vi "parse_binaries.vi"(4 "error in":errorcluster) -> (0 "error out":errorcluster)   [LabVIEW 2019]
doc: "Read and parse binary file according to the type of sensor. \nThis VI parse IMU, RPM , GPS, Camera and LiDAR binary files created with the mono_logger.vi"
uses:
  controls/radarSample.ctl
  controls/RadarTrack.ctl
panel:
  in  "JPEG":bool
  in  "Tab Control":enum32{"Camera", "GPS", "IMU/RPM", "Radar"}(tab)
  out "Camera":picture
  out "GPS":T1
  out "IMU":T2
  out "RPM":T3
  out "Radar Sample":T4
  in  "Sensor configuration":path
  out "Frame Number":i32
  in  "Save images to ...":path
  in  "VeloView port":u16=2368
  out "Sensor Type":string(combo)="gps"
  in  "stop":bool
  # "Only for LiDAR"
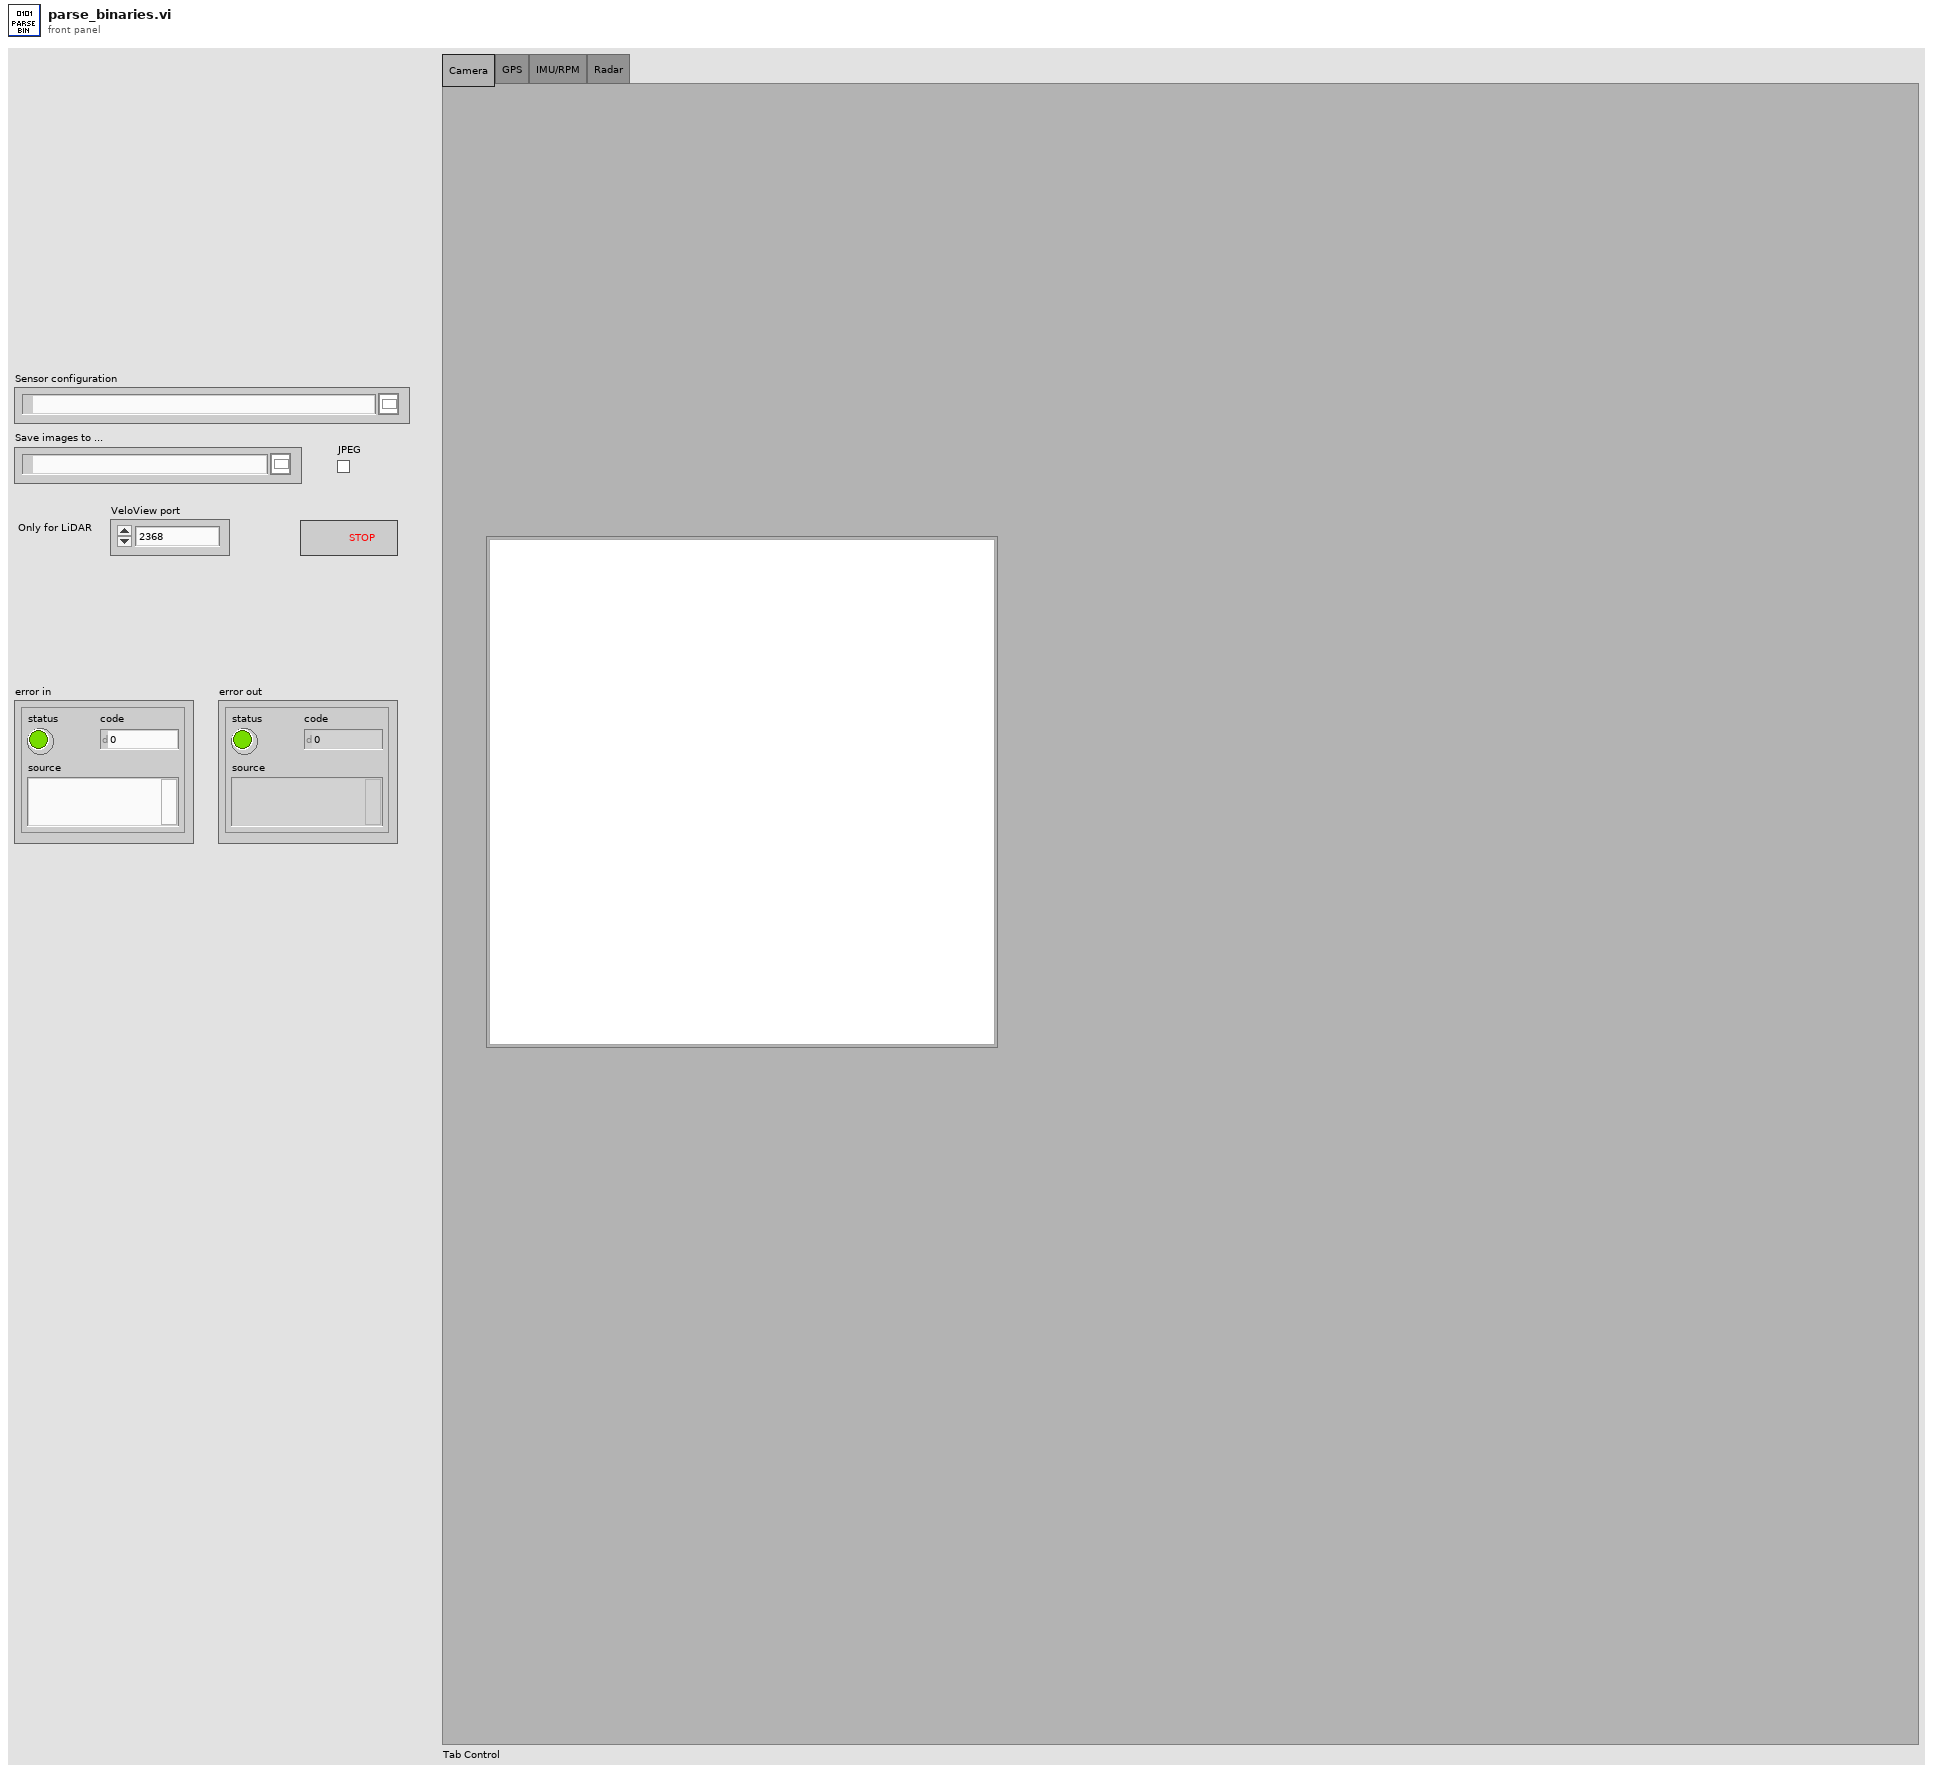
[diagram p1: front panel]
types:
  T1 = cluster{"preamble":u8, "MSG_POS_LLH":u16, "sensor_id":u16, "payload_length":u8, "latitude":dbl, "longitude":dbl, "elevation":dbl, "WorldLocation_x":sgl, "WorldLocation_y":sgl, "forward_x":sgl, "forward_y":sgl, "forward_z":sgl, "ego_yaw":sgl, "ego_speed":sgl, "horizontal_acceleration":u16, "vertical_acceleration":i16, "satellites":i8, "mode":i8, "CRC":i16}
  T2 = cluster{"packetSize":u8, "accel_x":sgl, "accel_y":sgl, "accel_z":sgl, "angle_rate_x":sgl, "angle_rate_y":sgl, "angle_rate_z":sgl, "timer":u32, "checksum":u16, "timeWeek":i32}
  T3 = cluster{"wheel_number":i32, "wheel_speed_lf":sgl}
  T4 = typedef "radarSample.ctl" = cluster{"Number of targets":i32, "gt_targets":cluster{"aoa":sgl, "range":sgl, "rcs":sgl, "velocity":sgl, "target_ids":string[]}[], "target_list":cluster{"aoa":sgl, "range":sgl, "rcs":sgl, "velocity":sgl, "target_ids":string[]}[], "tracks":T5[], "roi_targets":cluster{"roi_name":string, "radar_target":cluster{"aoa":sgl, "range":sgl, "rcs":sgl, "velocity":sgl, "target_ids":string[]}}[]}
  T5 = typedef "RadarTrack.ctl" = cluster{"track_id":u64, "x_range":sgl, "y_range":sgl, "heading":sgl, "velocity":sgl, "lifetime_seconds":sgl}
  T6 = enum16{"big-endian, network order", "native, host order", "little-endian"}
  T7 = enum16{"open", "replace", "create", "open or create", "replace or create", "replace or create with confirmation"}
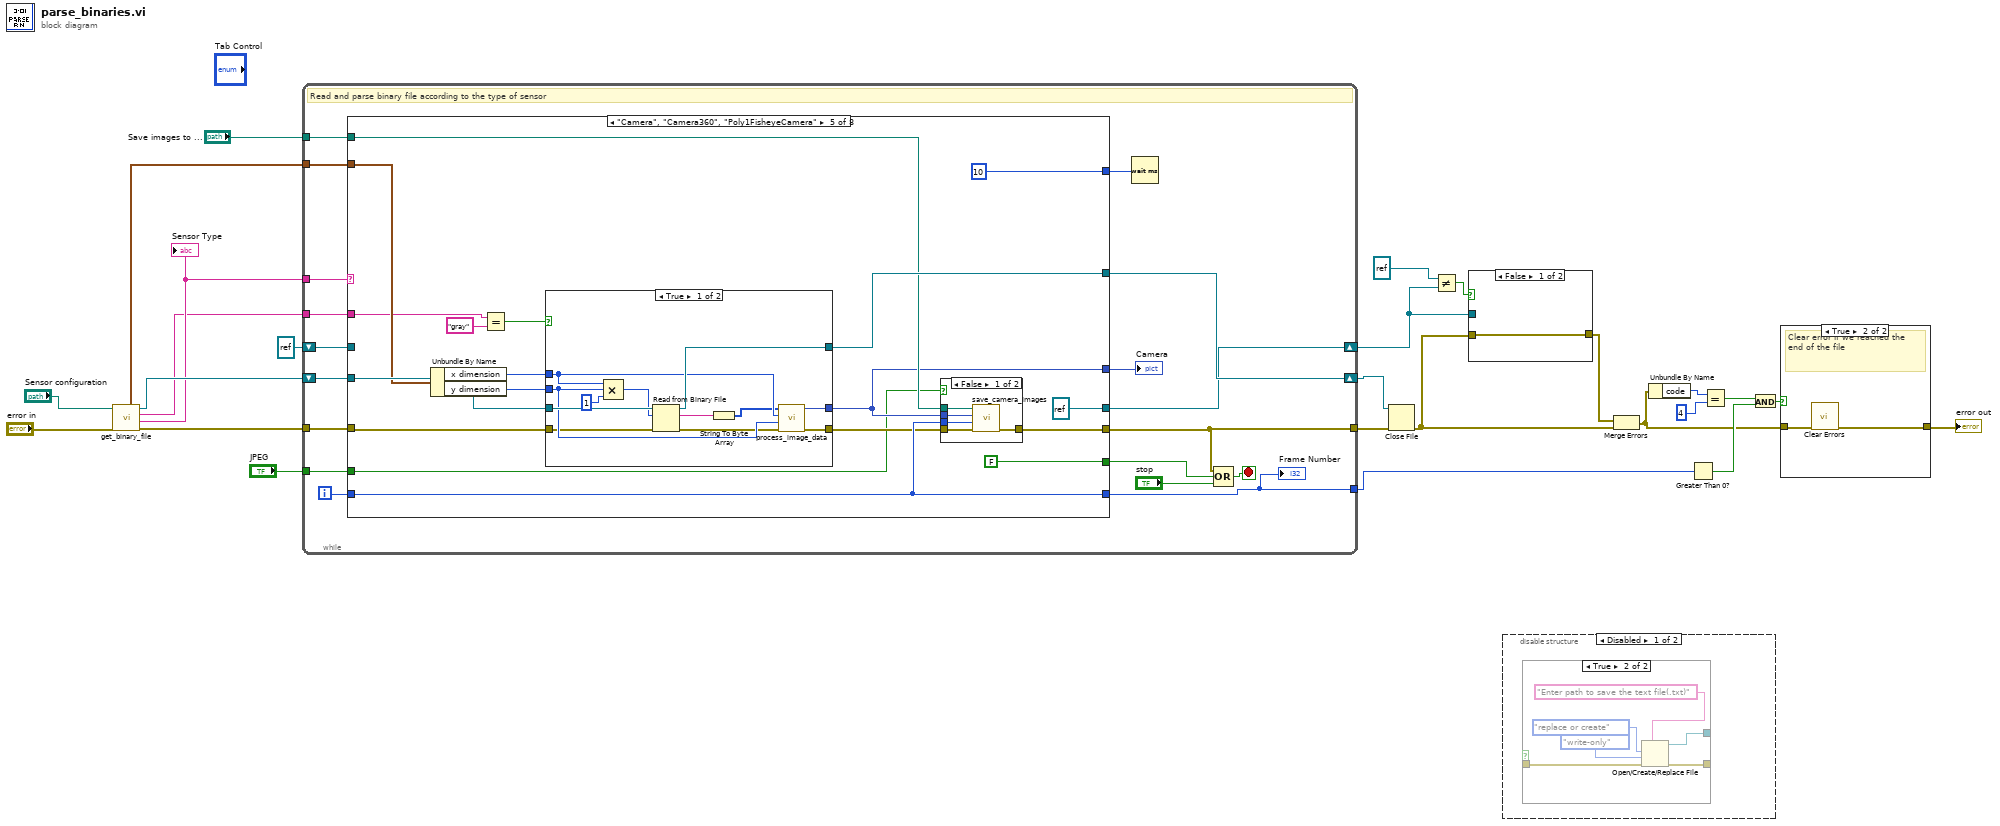
[diagram p0: block diagram]
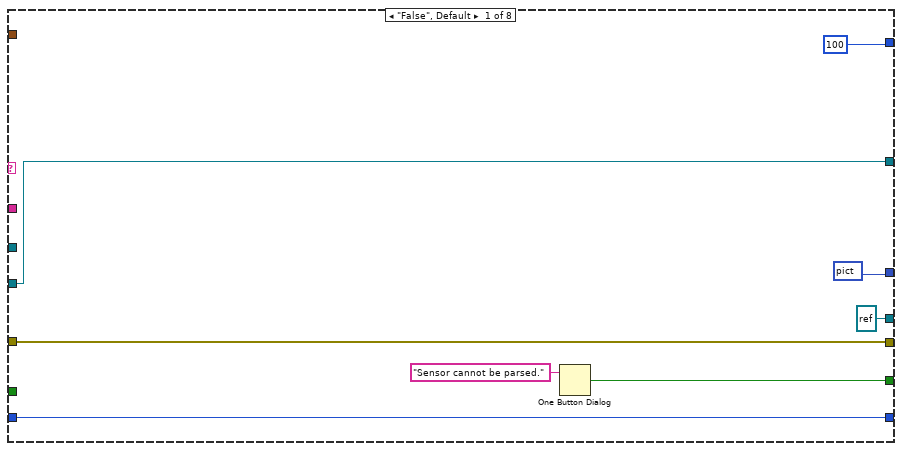
[diagram p2: hidden frame]
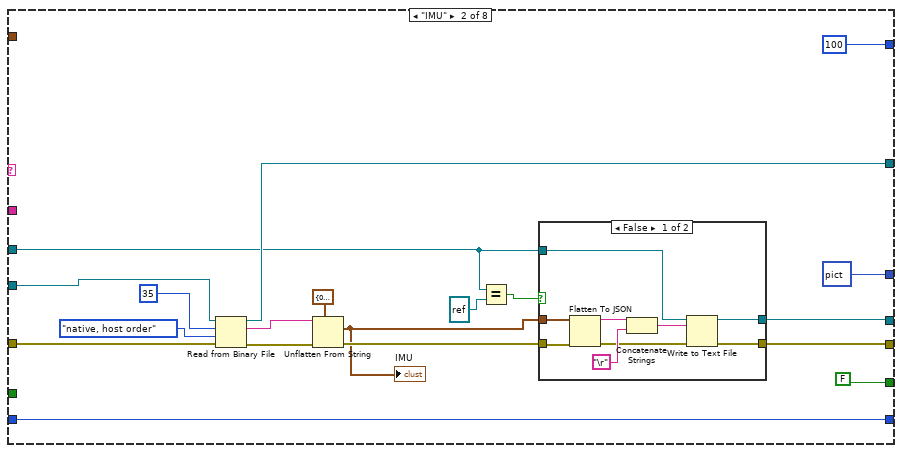
[diagram p3: hidden frame]
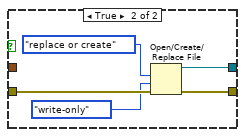
[diagram p4: hidden frame]
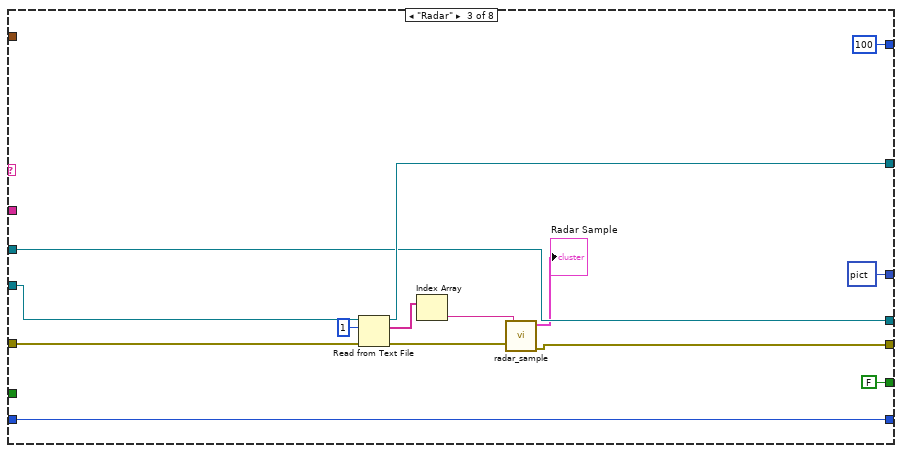
[diagram p5: hidden frame]
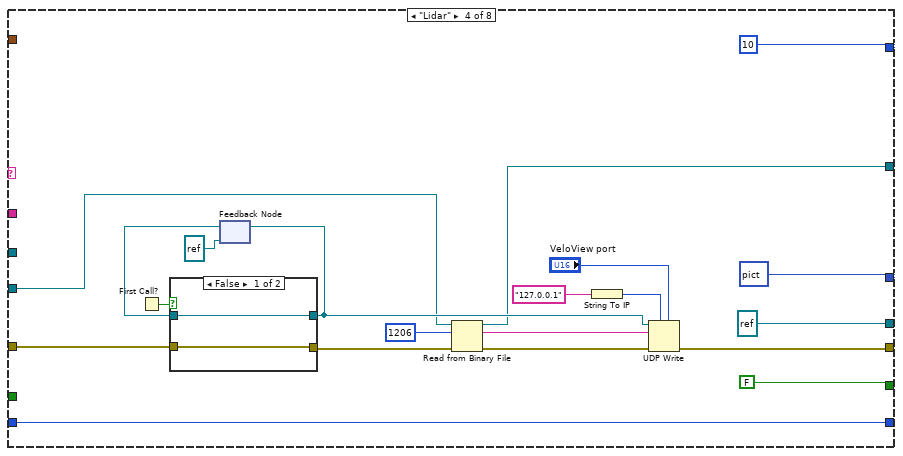
[diagram p6: hidden frame]
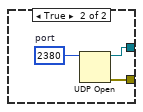
[diagram p7: hidden frame]
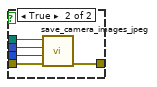
[diagram p8: hidden frame]
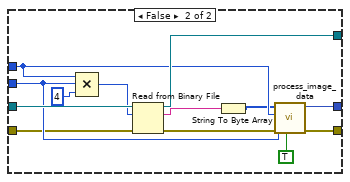
[diagram p9: hidden frame]
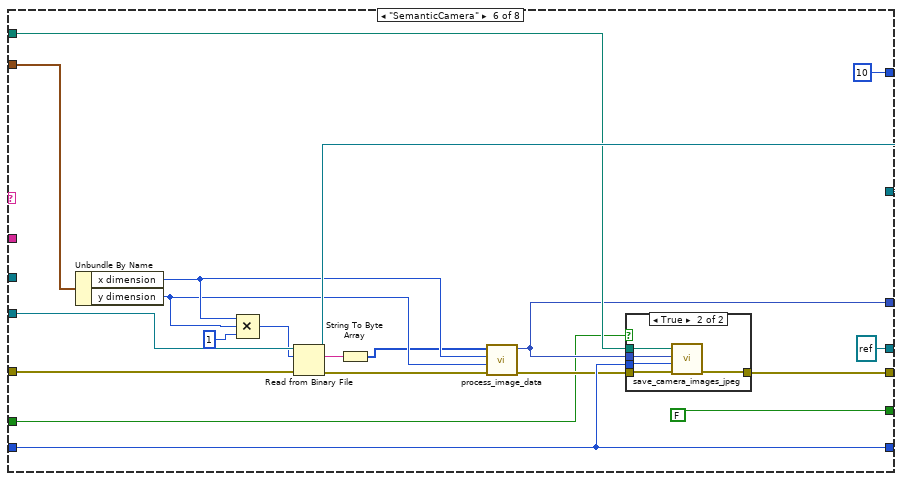
[diagram p10: hidden frame]
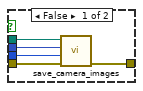
[diagram p11: hidden frame]
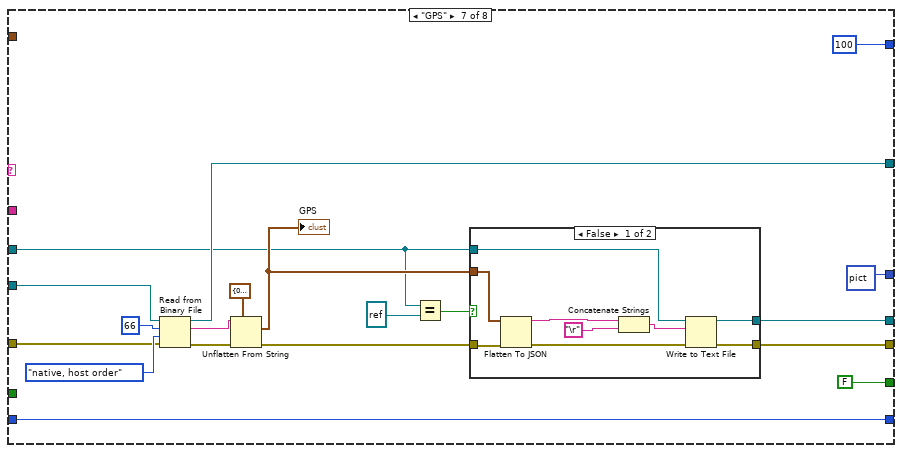
[diagram p12: hidden frame]
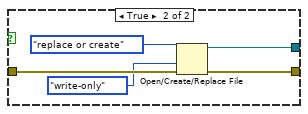
[diagram p13: hidden frame]
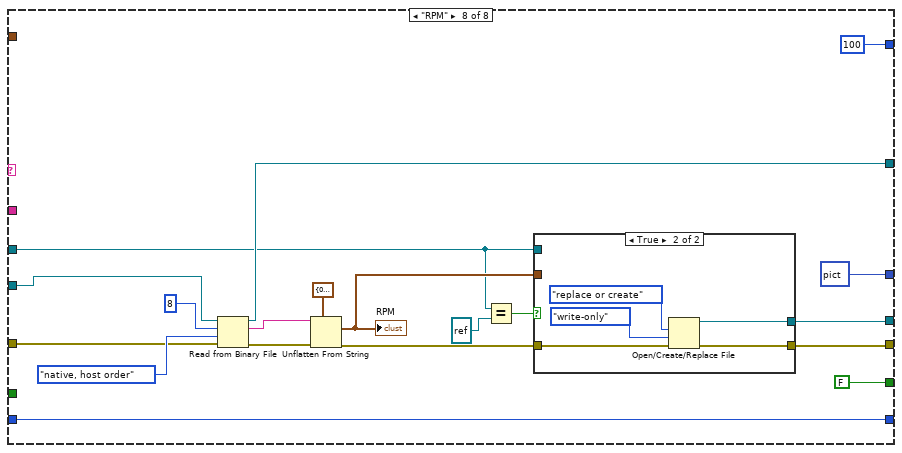
[diagram p14: hidden frame]
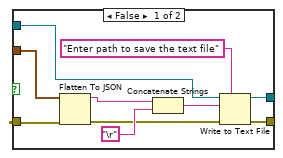
[diagram p15: hidden frame]
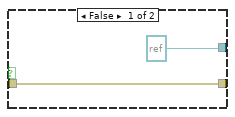
[diagram p16: hidden frame]
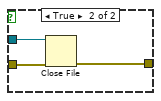
[diagram p19: hidden frame]
diagram:
  n1 = call "get_binary_file.vi"("error in"="error in", "Sensor configuration"="Sensor configuration") -> ("error out"=w21:errorcluster, "Type"=w11:string, "Channels"=w6:string, "Binary File ref"=w25:refnum<file>, "Stream dimensions"=w7:cluster{"x dimension":i32, "y dimension":i32})  [unwired: 5 in]
  "Sensor Type" <- w11
  n2 = while {
    shift-right: [w41] -> w24
    shift-left: w25 -> [w42]
    tunnel: [w34] -> w23
    tunnel: "Save images to ..." -> [w38]
    tunnel: w7 -> [w37]
    tunnel: w21 -> [w36]
    tunnel: [w33] -> w14
    tunnel: w11 -> [w32]
    tunnel: w6 -> [w28]
    shift-right: [w35] -> w19
    shift-left: refnum<file> refnum ("refnum out") -> [w27]
    tunnel: "JPEG" -> [w26]
    i -> [w39]
    stop <- w43 stop-if-true
    # "Read and parse binary file according to the type of sensor"
    n3 = case shown="\"Camera\", \"Camera360\", \"Poly1FisheyeCamera\"" w32 {
      tunnel: [w49 w57 w91 w113 w138 w191 w217 w246] -> w34
      tunnel: w42 -> [w51 w67 w96 w107 w141 w196 w221 w255]
      tunnel: [w51 w65 w89 w106 w140 w195 w220 w254] -> w41
      tunnel: [u32 100 ("milliseconds to wait") u32 100 ("milliseconds to wait") u32 100 ("milliseconds to wait") u32 10 ("milliseconds to wait") u32 10 ("milliseconds to wait") u32 10 ("milliseconds to wait") u32 100 ("milliseconds to wait") u32 100 ("milliseconds to wait")] -> w40
      tunnel: w39 -> [w48 w62 w98 w102 w135 w188 w211 w250]
      tunnel: w38 -> [_ _ _ _ w137 w190 _ _]
      tunnel: w37 -> [_ _ _ _ w136 w189 _ _]
      tunnel: w36 -> [w49 w53 w97 w103 w130 w186 w208 w241]
      tunnel: [refnum<file> refnum ("refnum out") w56 w87 refnum<file> refnum ("refnum out") refnum<file> refnum ("refnum out") refnum<file> refnum ("refnum out") w214 w245] -> w35
      tunnel: [w48 w62 w98 w102 w135 w188 w211 w250] -> w33
      tunnel: [picture data[5B] ("new picture") picture data[5B] ("new picture") picture data[5B] ("new picture") picture data[5B] ("new picture") w131 w183 picture data[5B] ("new picture") picture data[5B] ("new picture")] -> w31
      tunnel: [w45 FALSE ("true") FALSE ("true") FALSE ("true") FALSE ("true") FALSE ("true") FALSE ("true") FALSE ("true")] -> w29
      tunnel: w28 -> [_ _ _ _ w128 _ _ _]
      tunnel: w27 -> [_ w52 w87 _ _ _ w207 w240]
      tunnel: w26 -> [_ _ _ _ w124 w177 _ _]
      frame "False", Default {
        n4 = One Button Dialog(message="Sensor cannot be parsed.") -> (true=w45:bool)  [unwired: 1 in]
      }
      frame "IMU" {
        n5 = Read from Binary File(8:w53, 9:T6."native, host order" ("byte order (0:big-endian, network order)"), 10:35 ("count (1)"), 11:w67) -> (0:w66:errorcluster, 2:w64:string, 3:w65:refnum<file>)  [unwired: 2 in, 1 out]
        n6 = Unflatten From String(type=T2 {"packetSize"=0, "accel_x"=0.0, "accel_y"=0.0, "accel_z"=0.0, "angle_rate_x"=0.0, "angle_rate_y"=0.0, "angle_rate_z"=0.0, "timer"=0, "checksum"=0, "timeWeek"=0} ("IMU Data format"), binary string=w64, error in (no error)=w66) -> (value=w58:T2, error out=w59:errorcluster)  [unwired: 2 in, 1 out]
        "IMU" <- w58
        n7 = Equal?(x=w52, y=refnum<file> refnum ("refnum out")) -> (x = y?=w60:bool)
        n8 = case shown="False" w60 {
          tunnel: [w79 w83] -> w57
          tunnel: w58 -> [w78 _]
          tunnel: w59 -> [w77 w84]
          tunnel: [w72 w80] -> w56
          tunnel: w52 -> [w71 _]
          frame False {
            n9 = Flatten To JSON(anything=w78, error in (no error)=w77) -> (JSON string=w74:string, 11:w73:errorcluster)  [unwired: 1 in]
            n10 = Concatenate Strings(w74, "\r") -> (w76:string)
            n11 = Write to Text File(file (use dialog)=w71, text=w76, error in=w73) -> (refnum out=w72:refnum<file>, error out=w79:errorcluster)  [unwired: 1 in, 1 out]
          }
          frame True {
            n12 = Open/Create/Replace File(error in=w84, operation (0:open)=T7."replace or create", access (0:read/write)=enum16{"read/write", "read-only", "write-only"}."write-only") -> (refnum out=w80:refnum<file>, error out=w83:errorcluster)  [unwired: 3 in, 1 out]
          }
        }
      }
      frame "Radar" {
        n13 = Read from Text File(file (use dialog)=w96, count=1, error in=w97) -> (refnum out=w89:refnum<file>, text=w93:string[], error out=w94:errorcluster)  [unwired: 1 in, 1 out]
        n14 = Index Array(array=w93) -> (element=w92:string)  [unwired: 1 in]
        n15 = call "radar_sample.vi"("error in"=w94, "Raw data"=w92) -> ("error out"=w91:errorcluster, "Radar Sample"=→"Radar Sample":T4)  [unwired: 4 in]
      }
      frame "Lidar" {
        n16 = First Call?() -> (First Call?: T/F=w112:bool)
        n17 = feedback #1(refnum<k16> refnum ("port")) -> (w110:refnum<k16>)
        n18 = case shown="False" w112 {
          tunnel: [w119 w122] -> w111
          tunnel: [w120 w121] -> w109
          tunnel: w110 -> [w120 _]
          tunnel: w103 -> [w119 _]
          frame False {
          }
          frame True {
            w123 = u16 2380  # port
            n19 = UDP Open(11:w123) -> (port=w121:refnum<k16>, 0:w122:errorcluster)  [unwired: 4 in, 1 out]
          }
        }
        n20 = feedback-in #1(w109) -> ()
        n21 = Read from Binary File(8:w111, 10:1206 ("count (1)"), 11:w107) -> (0:w117:errorcluster, 2:w108:string, 3:w106:refnum<file>)  [unwired: 3 in, 1 out]
        n22 = String To IP(1:"127.0.0.1" ("veloview address input")) -> (0:w115:u32)
        n23 = UDP Write(address=w115, port or service name="VeloView port", connection ID=w109, data in=w108, 8:w117) -> (error out=w113:errorcluster)  [unwired: 1 in, 1 out]
      }
      frame "Camera", "Camera360", "Poly1FisheyeCamera" {
        n24 = Unbundle By Name(w136) -> ("x dimension"=w134:i32, "y dimension"=w133:i32)
        n25 = Equal?(x=w128, y="gray") -> (x = y?=w126:bool)
        n26 = case shown="True" w126 {
          tunnel: w141 -> [w163 w176]
          tunnel: [w162 w175] -> w140
          tunnel: w134 -> [w158 w171]
          tunnel: w133 -> [w157 w170]
          tunnel: [w155 w168] -> w132
          tunnel: [w154 w167] -> w131
          tunnel: w130 -> [w153 w166]
          frame True {
            n27 = Compound Arithmetic op=MULTIPLY(w158, w157, 1 ("value")) -> (w160:i32)
            n28 = Read from Binary File(8:w153, 10:w160, 11:w163) -> (0:w156:errorcluster, 2:w161:string, 3:w162:refnum<file>)  [unwired: 3 in, 1 out]
            n29 = String To Byte Array(string=w161) -> (unsigned byte array=w152:u8[])
            n30 = call "process_image_data.vi"("error in"=w156, "y"=w157, "x"=w158, "Raw data"=w152) -> ("error out"=w155:errorcluster, "Image"=w154:picture)  [unwired: 4 in]
          }
          frame False {
            n31 = Compound Arithmetic op=MULTIPLY(w171, w170, 4 ("value")) -> (w173:i32)
            n32 = Read from Binary File(8:w166, 10:w173, 11:w176) -> (0:w169:errorcluster, 2:w174:string, 3:w175:refnum<file>)  [unwired: 3 in, 1 out]
            n33 = String To Byte Array(string=w174) -> (unsigned byte array=w164:u8[])
            n34 = call "process_image_data.vi"("RGBA"=TRUE, "error in"=w169, "y"=w170, "x"=w171, "Raw data"=w164) -> ("error out"=w168:errorcluster, "Image"=w167:picture)  [unwired: 3 in]
          }
        }
        n35 = case shown="False" w124 {
          tunnel: [w146 w151] -> w138
          tunnel: w137 -> [w145 w147]
          tunnel: w135 -> [w144 w149]
          tunnel: w132 -> [w143 w150]
          tunnel: w131 -> [w142 w148]
          frame False {
            n36 = call "save_camera_images.vi"("error in"=w143, "frame_number"=w144, "Image"=w142, "Path to save image"=w145) -> ("error out"=w146:errorcluster)  [unwired: 3 in]
          }
          frame True {
            n37 = call "save_camera_images_jpeg.vi"("error in"=w150, "frame_number"=w149, "Image"=w148, "Path to save image"=w147) -> ("error out"=w151:errorcluster)  [unwired: 3 in]
          }
        }
      }
      frame "SemanticCamera" {
        n38 = Unbundle By Name(w189) -> ("x dimension"=w182:i32, "y dimension"=w181:i32)
        n39 = Compound Arithmetic op=MULTIPLY(w182, w181, 1 ("value")) -> (w192:i32)
        n40 = Read from Binary File(8:w186, 10:w192, 11:w196) -> (0:w185:errorcluster, 2:w193:string, 3:w195:refnum<file>)  [unwired: 3 in, 1 out]
        n41 = String To Byte Array(string=w193) -> (unsigned byte array=w179:u8[])
        n42 = call "process_image_data.vi"("error in"=w185, "y"=w181, "x"=w182, "Raw data"=w179) -> ("error out"=w184:errorcluster, "Image"=w183:picture)  [unwired: 4 in]
        n43 = case shown="True" w177 {
          tunnel: [w201 w205] -> w191
          tunnel: w190 -> [w200 w204]
          tunnel: w188 -> [w199 w202]
          tunnel: w184 -> [w198 w206]
          tunnel: w183 -> [w197 w203]
          frame False {
            n44 = call "save_camera_images.vi"("error in"=w198, "frame_number"=w199, "Image"=w197, "Path to save image"=w200) -> ("error out"=w201:errorcluster)  [unwired: 3 in]
          }
          frame True {
            n45 = call "save_camera_images_jpeg.vi"("error in"=w206, "frame_number"=w202, "Image"=w203, "Path to save image"=w204) -> ("error out"=w205:errorcluster)  [unwired: 3 in]
          }
        }
      }
      frame "GPS" {
        n46 = Read from Binary File(8:w208, 9:T6."native, host order" ("byte order (0:big-endian, network order)"), 10:66 ("count (1)"), 11:w221) -> (0:w222:errorcluster, 2:w219:string, 3:w220:refnum<file>)  [unwired: 2 in, 1 out]
        n47 = Unflatten From String(type=T1 {"preamble"=0, "MSG_POS_LLH"=0, "sensor_id"=0, "payload_length"=0, "latitude"=0.0, "longitude"=0.0, "elevation"=0.0, "WorldLocation_x"=0.0, "WorldLocation_y"=0.0, "forward_x"=0.0, "forward_y"=0.0, "forward_z"=0.0, "ego_yaw"=0.0, "ego_speed"=0.0, "horizontal_acceleration"=0, "vertical_acceleration"=0, "satellites"=0, "mode"=0, "CRC"=0} ("gps format"), binary string=w219, error in (no error)=w222) -> (value=w216:T1, error out=w215:errorcluster)  [unwired: 2 in, 1 out]
        "GPS" <- w216
        n48 = Equal?(x=w207, y=refnum<file> refnum ("refnum out")) -> (x = y?=w212:bool)
        n49 = case shown="False" w212 {
          tunnel: [w234 w238] -> w217
          tunnel: w216 -> [w233 _]
          tunnel: w215 -> [w232 w239]
          tunnel: [w227 w235] -> w214
          tunnel: w207 -> [w226 _]
          frame False {
            n50 = Flatten To JSON(anything=w233, error in (no error)=w232) -> (JSON string=w229:string, 11:w228:errorcluster)  [unwired: 1 in]
            n51 = Concatenate Strings(w229, "\r") -> (w231:string)
            n52 = Write to Text File(file (use dialog)=w226, text=w231, error in=w228) -> (refnum out=w227:refnum<file>, error out=w234:errorcluster)  [unwired: 1 in, 1 out]
          }
          frame True {
            n53 = Open/Create/Replace File(error in=w239, operation (0:open)=T7."replace or create", access (0:read/write)=enum16{"read/write", "read-only", "write-only"}."write-only") -> (refnum out=w235:refnum<file>, error out=w238:errorcluster)  [unwired: 3 in, 1 out]
          }
        }
      }
      frame "RPM" {
        n54 = Read from Binary File(8:w241, 9:T6."native, host order" ("byte order (0:big-endian, network order)"), 10:8 ("count (1)"), 11:w255) -> (0:w253:errorcluster, 2:w252:string, 3:w254:refnum<file>)  [unwired: 2 in, 1 out]
        n55 = Unflatten From String(type=T3 {"wheel_number"=0, "wheel_speed_lf"=0.0} ("rpm"), binary string=w252, error in (no error)=w253) -> (value=w244:T3, error out=w247:errorcluster)  [unwired: 2 in, 1 out]
        "RPM" <- w244
        n56 = Equal?(x=w240, y=refnum<file> refnum ("refnum out")) -> (x = y?=w248:bool)
        n57 = case shown="True" w248 {
          tunnel: [w268 w272] -> w246
          tunnel: w247 -> [w267 w273]
          tunnel: [w262 w269] -> w245
          tunnel: w244 -> [w261 _]
          tunnel: w240 -> [w259 _]
          frame False {
            n58 = Flatten To JSON(anything=w261, error in (no error)=w267) -> (JSON string=w264:string, 11:w263:errorcluster)  [unwired: 1 in]
            n59 = Concatenate Strings(w264, "\r") -> (w266:string)
            n60 = Write to Text File(prompt (Choose or enter file path)="Enter path to save the text file", file (use dialog)=w259, text=w266, error in=w263) -> (refnum out=w262:refnum<file>, error out=w268:errorcluster)  [unwired: 1 out]
          }
          frame True {
            n61 = Open/Create/Replace File(error in=w273, operation (0:open)=T7."replace or create", access (0:read/write)=enum16{"read/write", "read-only", "write-only"}."write-only") -> (refnum out=w269:refnum<file>, error out=w272:errorcluster)  [unwired: 3 in, 1 out]
          }
        }
      }
    }
    "Camera" <- w31
    "Frame Number" <- w33
    n62 = Wait (ms)(milliseconds to wait=w40) -> ()  [unwired: 1 out]
    n63 = Compound Arithmetic op=OR(w34, w29, "stop") -> (w43:bool)
  }
  n64 = Close File(refnum=w24, error in=w23) -> (error out=w4:errorcluster)  [unwired: 1 out]
  n65 = Not Equal?(x=refnum<file> refnum ("refnum out"), y=w19) -> (x != y?=w20:bool)
  n66 = case shown="False" w20 {
    tunnel: w4 -> [w274 w277]
    tunnel: w19 -> [_ w276]
    tunnel: [w274 w275] -> w2
    frame False {
    }
    frame True {
      n67 = Close File(refnum=w276, error in=w277) -> (error out=w275:errorcluster)  [unwired: 1 out]
    }
  }
  n68 = disable-structure shown="Disabled" {
    frame Disabled {
      n69 = case shown="True" {
        selector: _ -> [_ _]
        tunnel: _ -> [w279 w283]
        tunnel: [w279 w282] -> _
        tunnel: [refnum<file> refnum ("refnum out") w281] -> _
        frame False {
        }
        frame True {
          n70 = Open/Create/Replace File(error in=w283, prompt="Enter path to save the text file(.txt)" ("prompt (Choose or enter file path)"), operation (0:open)=T7."replace or create", access (0:read/write)=enum16{"read/write", "read-only", "write-only"}."write-only") -> (refnum out=w281:refnum<file>, error out=w282:errorcluster)  [unwired: 2 in, 1 out]
        }
      }
    }
    frame Enabled {
    }
  }
  n71 = Merge Errors(w2, w4) -> (w3:errorcluster)
  n72 = Unbundle By Name(w3) -> ("code"=w17:i32)
  n73 = Greater Than 0?(x=w14) -> (x > 0?=w12:bool)
  n74 = Equal?(x=w17, y=4) -> (x = y?=w13:bool)
  n75 = And(x=w13, y=w12) -> (x .and. y?=w15:bool)
  n76 = case shown="True" w15 {
    tunnel: w3 -> [w286 w288]
    tunnel: [w286 w287] -> w10
    frame False {
      # "Error 4, indicate empty file"
    }
    frame True {
      # "Clear error if we reached the end of the file"
      n77 = call <vilib>:"Clear Errors.vi"("error in (no error)"=w288) -> ("error out"=w287:errorcluster)  [unwired: 5 in, 1 out]
    }
  }
  "error out" <- w10
